vi "File.Async Mover_v2.vi"(9 "Error Msg":T1={"Cmd"="Task", "Sub"="Warning", "Data1"=variant, "Data2"=variant}, 10 "Parent Q":refnum<queue>, 11 "Q Name":string="FileMover") -> ()   [LabVIEW 2018]
uses:
  <vilib>/KATE/Queues/Q.Element.ctl
  File.Async Mover Move Task Item.ctl
  <vilib>/KATE/Queues/Queue Utils.lvlib
  <vilib>/KATE/Files/File Utils.lvlib
  <vilib>/KATE/Scheduler/Scheduler.lvlib
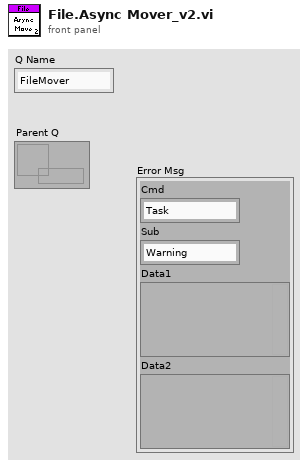
[diagram p1: front panel]
types:
  T1 = typedef "KATE_Lib.lvlib/Queue Utils.lvlib/Q.Element.ctl" = cluster{"Cmd":string, "Sub":string, "Data1":variant, "Data2":variant}
  T2 = typedef "File.Async Mover Move Task Item.ctl" = cluster{"Source":path, "DestDir":path, "DestSuffix":string, "Action":enum16{"Move", "Copy"}}
  T3 = cluster{"TempDir":path, "TaskDir":path, "Tasks":T2[]}
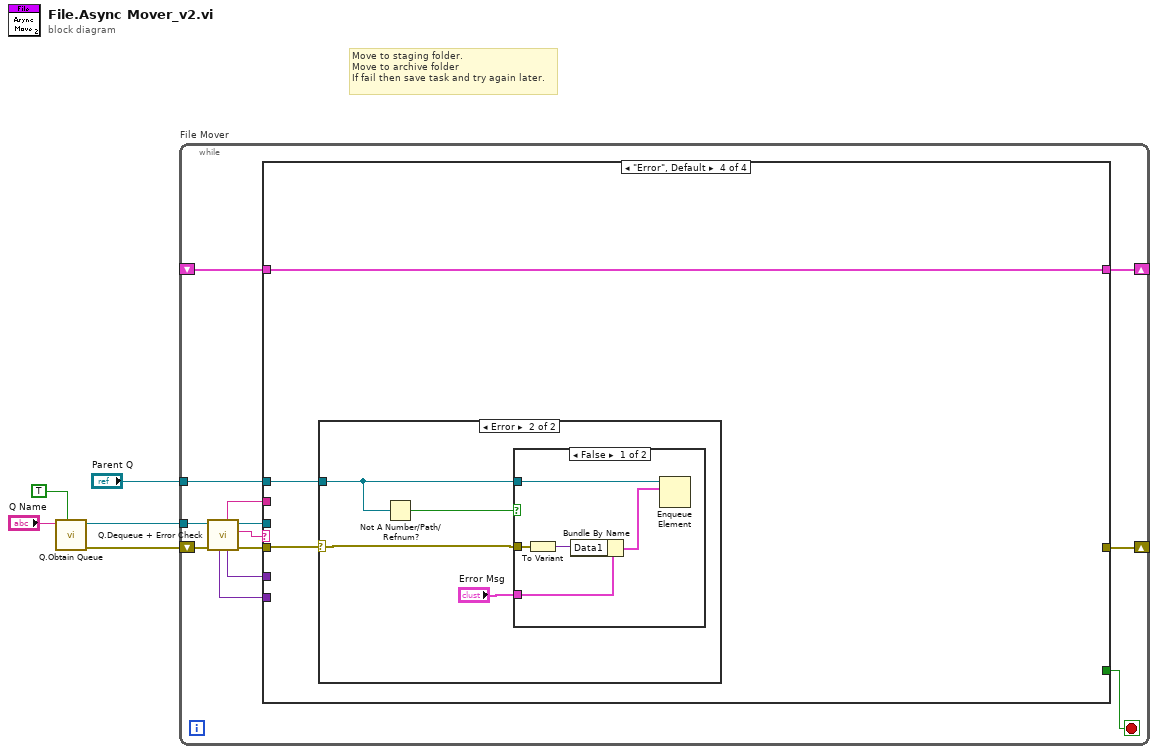
[diagram p0: block diagram]
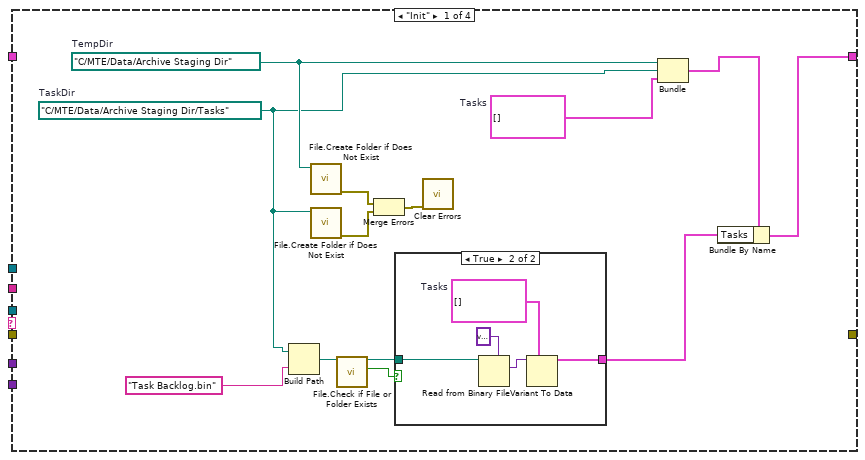
[diagram p2: hidden frame]
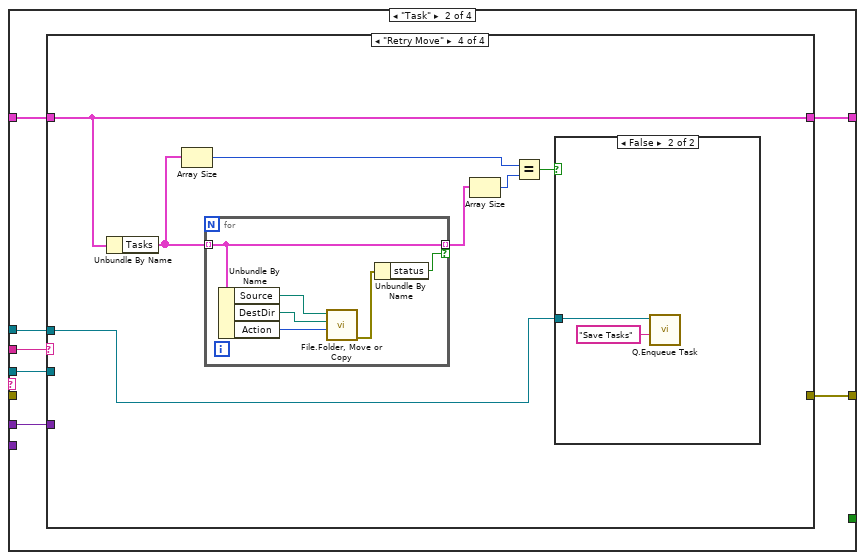
[diagram p4: hidden frame]
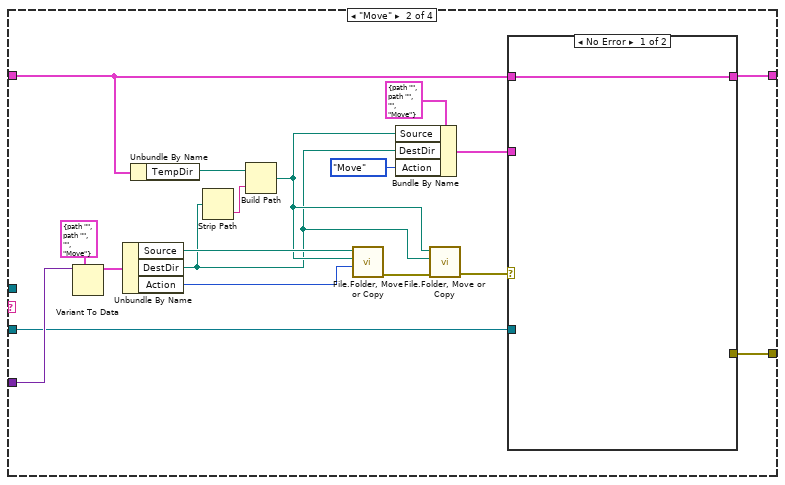
[diagram p6: hidden frame]
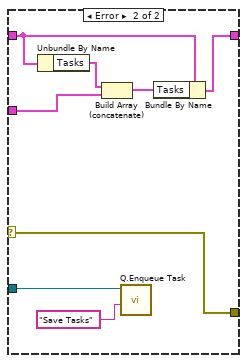
[diagram p7: hidden frame]
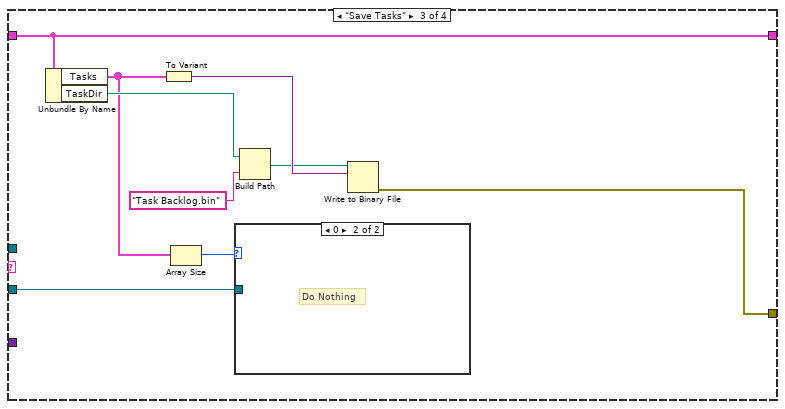
[diagram p8: hidden frame]
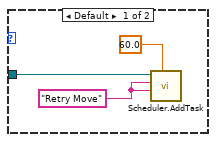
[diagram p9: hidden frame]
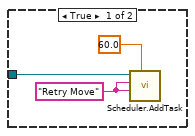
[diagram p10: hidden frame]
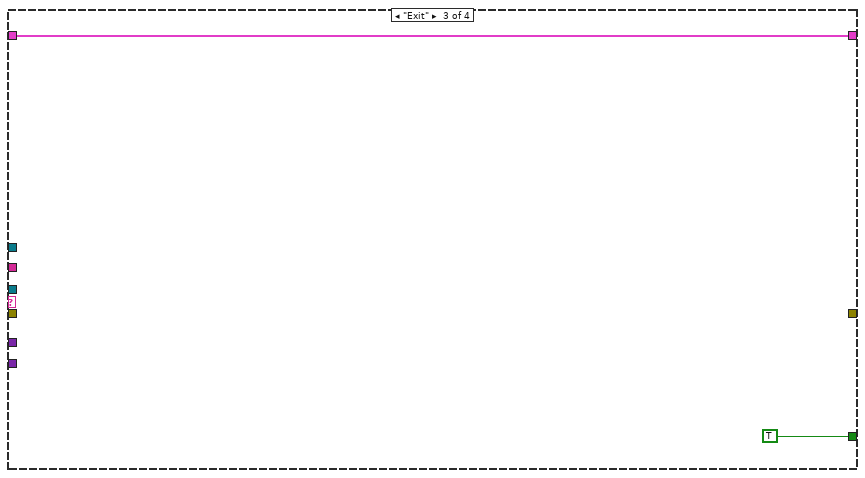
[diagram p11: hidden frame]
diagram:
  # "Move to staging folder.\nMove to archive folder\nIf fail then save task and try again later."
  n1 = call <vilib>:"Q.Obtain Queue.vi"("Enqueue Init"=TRUE, "Q Name"="Q Name") -> ("error out"=w5:errorcluster, "Q Out"=w4:refnum<queue>)  [unwired: 7 in, 1 out]
  n2 = while "File Mover" {
    tunnel: w4 -> [w18]
    shift-right: [w13] -> _
    shift-left: w5 -> [w17]
    tunnel: "Parent Q" -> [w11]
    shift-right: [w7] -> _
    shift-left: _ -> [w6]
    stop <- w10 stop-if-true
    n3 = call <vilib>:"Q.Dequeue + Error Check.vi"("Error In"=w17, "Q In"=w18) -> ("error out"=w9:errorcluster, "Cmd"=w12:string, "Q Out"=w16:refnum<queue>, "Data1"=w15:variant, "Sub"=w8:string, "Data2"=w14:variant)  [unwired: 4 in]
    n4 = case shown="\"Error\", Default" w12 {
      tunnel: w16 -> [_ w39 _ _]
      tunnel: w15 -> [_ w43 _ _]
      tunnel: w14 -> [_ _ _ _]
      tunnel: [_ w42 _ _] -> w13
      tunnel: w11 -> [_ w40 _ w105]
      tunnel: [_ _ TRUE _] -> w10
      tunnel: w9 -> [_ _ _ w106]
      tunnel: w8 -> [_ w41 _ _]
      tunnel: [w22 w37 w102 w104] -> w7
      tunnel: w6 -> [_ w38 w102 w104]
      frame "Init" {
        w27 = T2[] []  # Tasks
        w24 = path "C:/MTE/Data/Archive Staging Dir/Tasks"  # TaskDir
        w31 = path "C:/MTE/Data/Archive Staging Dir"  # TempDir
        n5 = Build Path(base path=w24, name or relative path="Task Backlog.bin") -> (appended path=w21:path)
        n6 = call <vilib>:"File.Create Folder if Does Not Exist.vi"("Path"=w31) -> ("error out"=w30:errorcluster)  [unwired: 8 in, 2 out]
        n7 = call <vilib>:"File.Create Folder if Does Not Exist.vi"("Path"=w24) -> ("error out"=w29:errorcluster)  [unwired: 8 in, 2 out]
        n8 = call <vilib>:"File.Check if File or Folder Exists.vi"("Path"=w21) -> ("Exists"=w19:bool, "Dup Path"=w20:path)  [unwired: 6 in, 3 out]
        n9 = Merge Errors(w30, w29) -> (w28:errorcluster)
        n10 = case shown="True" w19 {
          tunnel: w20 -> [_ w36]
          tunnel: [_ w35] -> w25
          frame False {
          }
          frame True {
            w34 = T2[] []  # Tasks
            n11 = Read from Binary File(5:variant ("variant"), 11:w36) -> (2:w32:variant)  [unwired: 4 in, 3 out]
            n12 = Variant To Data(type=w34, Variant=w32) -> (data=w35:T2[])  [unwired: 1 in, 1 out]
          }
        }
        n13 = call <vilib>:"Clear Errors.vi"("error in (no error)"=w28) -> ()  [unwired: 5 in, 2 out]
        n14 = Bundle("TempDir"=w31, "TaskDir"=w24, "Tasks"=w27) -> (w23:T3)  [unwired: 1 in]
        n15 = Bundle By Name(cluster=w23, "Tasks"=w25) -> (w22:T3)
      }
      frame "Task" {
        n16 = case shown="\"Retry Move\"" w41 {
          tunnel: w43 -> [_ w62 _ _]
          tunnel: [_ w45 w76 _] -> w42
          tunnel: w40 -> [_ _ _ w88]
          tunnel: w39 -> [_ w46 w74 _]
          tunnel: w38 -> [w44 w50 w75 w90]
          tunnel: [w44 w47 w75 w90] -> w37
          frame Default {
          }
          frame "Move" {
            n17 = Variant To Data(type=T2 {"Source"=path "", "DestDir"=path "", "DestSuffix"="", "Action"=enum."Move"} ("cluster"), Variant=w62) -> (data=w61:T2)  [unwired: 1 in, 1 out]
            n18 = Unbundle By Name(w61) -> ("Source"=w59:path, "DestDir"=w51:path, "Action"=w58:enum16{"Move", "Copy"})
            n19 = Unbundle By Name(w50) -> ("TempDir"=w56:path)
            n20 = Strip Path(path=w51) -> (name=w54:string)  [unwired: 1 out]
            n21 = Build Path(base path=w56, name or relative path=w54) -> (appended path=w52:path)
            n22 = call "File.Folder, Move or Copy.vi"("Action"=w58, "Dest"=w52, "Source"=w59) -> ("error out"=w53:errorcluster)  [unwired: 7 in, 1 out]
            n23 = Bundle By Name(cluster=T2 {"Source"=path "", "DestDir"=path "", "DestSuffix"="", "Action"=enum."Move"}, "Source"=w52, "DestDir"=w51, "Action"=enum16{"Move", "Copy"}."Move") -> (w48:T2)
            n24 = call "File.Folder, Move or Copy.vi"("error in (no error)"=w53, "Dest"=w51, "Source"=w52) -> ("error out"=w49:errorcluster)  [unwired: 7 in, 1 out]
            n25 = case shown="No Error" w49 {
              selector: w49 -> [_ w64]
              tunnel: w50 -> [w63 w69]
              tunnel: w48 -> [_ w71]
              tunnel: [w63 w67] -> w47
              tunnel: w46 -> [_ w66]
              tunnel: [_ w64] -> w45
              frame No Error {
              }
              frame Error {
                n26 = Unbundle By Name(w69) -> ("Tasks"=w70:T2[])
                n27 = Build Array (concatenate)(w70, w71) -> (w68:T2[])
                n28 = call <vilib>:"Q.Enqueue Task.vi"("Task Name"="Save Tasks", "Q In"=w66) -> ()  [unwired: 8 in, 2 out]
                n29 = Bundle By Name(cluster=w69, "Tasks"=w68) -> (w67:T3)
              }
            }
          }
          frame "Save Tasks" {
            n30 = Unbundle By Name(w75) -> ("Tasks"=w73:T2[], "TaskDir"=w78:path)
            n31 = To Variant(anything=w73) -> (Variant=w80:variant)
            n32 = Array Size(array=w73) -> (size(s)=w72:i32)
            n33 = case shown="0" w72 {
              tunnel: w74 -> [w83 _]
              frame Default {
                w82 = "Retry Move" ("Sched Name")
                n34 = call <vilib>:"Scheduler.AddTask.vi"("Interval(s)"=60.0, "Task Name"=w82, "Sched Name"=w82, "Q In"=w83) -> ()  [unwired: 6 in, 2 out]
              }
              frame 0 {
                # "Do Nothing"
              }
            }
            n35 = Build Path(base path=w78, name or relative path="Task Backlog.bin") -> (appended path=w77:path)
            n36 = Write to Binary File(file (use dialog)=w77, data=w80) -> (error out=w76:errorcluster)  [unwired: 4 in, 2 out]
          }
          frame "Retry Move" {
            n37 = Unbundle By Name(w90) -> ("Tasks"=w87:T2[])
            n38 = Array Size(array=w87) -> (size(s)=w86:i32)
            n39 = for {
              tunnel: w87 -> [w98] mode=indexing
              tunnel: [w98] -> w89 mode=indexing if=w96
              n40 = Unbundle By Name(w98) -> ("Source"=w101:path, "DestDir"=w100:path, "Action"=w99:enum16{"Move", "Copy"})
              n41 = call "File.Folder, Move or Copy.vi"("Action"=w99, "Dest"=w100, "Source"=w101) -> ("error out"=w97:errorcluster)  [unwired: 7 in, 1 out]
              n42 = Unbundle By Name(w97) -> ("status"=w96:bool)
            }
            n43 = Array Size(array=w89) -> (size(s)=w85:i32)
            n44 = Equal?(x=w86, y=w85) -> (x = y?=w84:bool)
            n45 = case shown="False" w84 {
              tunnel: w88 -> [w91 w95]
              frame True {
                w93 = "Retry Move" ("Sched Name")
                n46 = call <vilib>:"Scheduler.AddTask.vi"("Interval(s)"=60.0, "Task Name"=w93, "Sched Name"=w93, "Q In"=w91) -> ()  [unwired: 6 in, 2 out]
              }
              frame False {
                n47 = call <vilib>:"Q.Enqueue Task.vi"("Task Name"="Save Tasks", "Q In"=w95) -> ()  [unwired: 8 in, 2 out]
              }
            }
          }
        }
      }
      frame "Exit" {
        (unwired) TRUE
      }
      frame "Error", Default {
        n48 = case shown="Error" w106 {
          selector: w106 -> [_ w107]
          tunnel: w105 -> [_ w109]
          frame No Error {
          }
          frame Error {
            n49 = Not A Number/Path/Refnum?(number/path/refnum=w109) -> (NaN/Path/Refnum?=w110:bool)
            n50 = case shown="False" w110 {
              tunnel: w109 -> [w115 _]
              tunnel: "Error Msg" -> [w114 _]
              tunnel: w107 -> [w111 _]
              frame False {
                n51 = To Variant(anything=w111) -> (Variant=w112:variant)
                n52 = Bundle By Name(cluster=w114, "Data1"=w112) -> (w113:T1)
                n53 = Enqueue Element(queue=w115, element=w113) -> ()  [unwired: 2 in, 3 out]
              }
              frame True {
              }
            }
          }
        }
      }
    }
  }
